vi "Ranger Dashboard.vi"() -> ()   [LabVIEW 2012, in "Party_Program.exe.lvrbt"]
doc: "This VI is designed to control TETRIX motors and visualize sensor data from your TETRIX Ranger Robot. Verify that your robot is configured as shown in the Schematic Editor. If you reconfigure your TETRIX Ranger Robot, change the ports in this VI and the Schematic Editor."
uses:
  Party_Program.exe.lvrbt
  <vilib>/NXT/Hardware/Plugins/Tetrix DC Motor/TetrixDCMotorAddress.ctl
  <vilib>/NXT/Block Support/NXT_InputPort.ctl
  <vilib>/NXT/Dual Mode Library/Display/drawText.vi
  <vilib>/NXT/Dual Mode Library/Sensors/Sonar_cm.vi
  <vilib>/NXT/Dual Mode Library/Sensors/Color_Detector.vi
  <vilib>/NXT/Dual Mode Library/Sensors/Touch_Pressed.vi
  <vilib>/NXT/NXTIO Xnodes/NXTIONodeSubVIs/TETRIX IO Move DC Motors.vi
  <vilib>/NXT/NXTIO Xnodes/NXTIONodeSubVIs/TETRIX IO Check Battery.vi
  <vilib>/NXT/NXTIO Xnodes/NXTIONodeSubVIs/TETRIX IO Stop DC Motors.vi
  <vilib>/NXT/NXTIO Xnodes/AddressXNode/NXTIOAddress.xnode
  <vilib>/NXT/NXTIO Xnodes/NXTIOXNode/NXTIO.xnode
  <vilib>/NXT/Subs/LVHSConnector.ctl
  <vilib>/NXT/LegoClasses/BrickReference/BrickReference.lvclass
panel:
  out "Yes / No":bool
  out "Detected Color":i16
  in  "Stop":bool
  out "TETRIX Battery Voltage":sgl(slide) scale=0.0..100.0
  in  "Right Wheel":i8(slide) scale=-100.0..100.0
  in  "Left Wheel":i8(slide) scale=-100.0..100.0
  out "Ultrasonic Sensor Data":i16(graph)
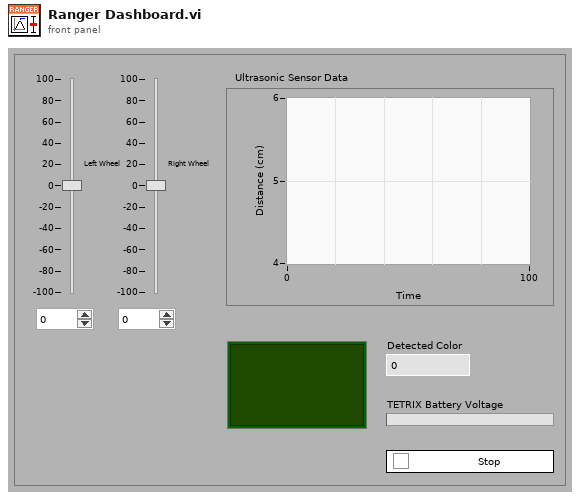
[diagram p1: front panel]
types:
  T1 = typedef "LVHSConnector.ctl" = refnum<class "BrickReference.lvclass">
  T2 = typedef "TetrixDCMotorAddress.ctl" = i16
  T3 = typedef "NXT_InputPort.ctl" = u8
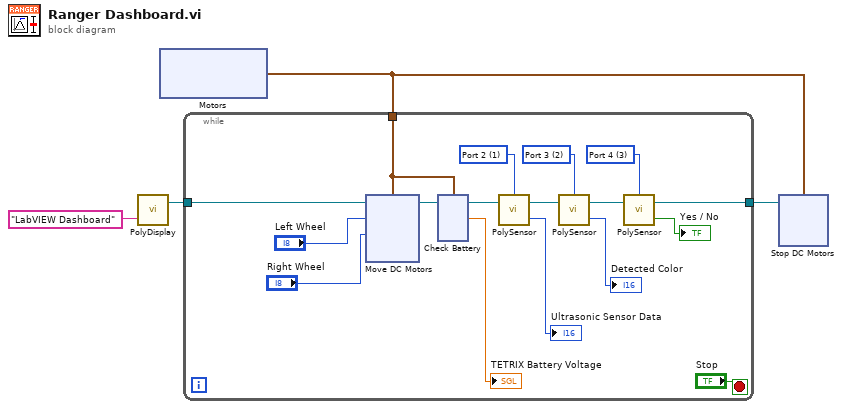
[diagram p0: block diagram]
diagram:
  n1 = call-poly <vilib>:"PolyDisplay.vi"("Text"="LabVIEW Dashboard") -> ("NXT"=w3:T1)  [unwired: 3 in]
  n2 = xnode "Motors"() -> ("Motor"=w2:cluster{"TetrixDCMotor":T2, "TetrixDCMotor":T2})
  n3 = while {
    tunnel: [w7] -> w4
    tunnel: w3 -> [w6]
    tunnel: w2 -> [w5]
    stop <- "Stop" stop-if-true
    w15 = T3 3 items=["Port 1", "Port 2", "Port 3", "Port 4"] ("Port (Port 4)")
    w16 = T3 2 items=["Port 1", "Port 2", "Port 3", "Port 4"] ("Port (Port 4)")
    w19 = T3 1 items=["Port 1", "Port 2", "Port 3", "Port 4"] ("Port (Port 4)")
    n4 = xnode "Move DC Motors"("Power/Speed 2"="Right Wheel", "Power/Speed 1"="Left Wheel", "Motors"=w5, "NXT"=w6) -> ("NXT"=w12:T1)
    n5 = xnode "Check Battery"("Motors"=w5, "NXT"=w12) -> ("Voltage 1"=→"TETRIX Battery Voltage":sgl, "NXT"=w10:T1)  [unwired: 1 out]
    n6 = call-poly <vilib>:"PolySensor.vi"("NXT"=w10, "Port (Port 4)"=w19) -> ("Distance (cm)"=→"Ultrasonic Sensor Data":i16, "NXT"=w9:T1)  [unwired: 1 in]
    n7 = call-poly <vilib>:"PolySensor.vi"("NXT"=w9, "Port (Port 3)"=w16) -> ("Detected Color"=→"Detected Color":i16, "NXT"=w8:T1)  [unwired: 1 in]
    n8 = call-poly <vilib>:"PolySensor.vi"("NXT"=w8, "Port (Port 1)"=w15) -> ("Yes / No"=→"Yes / No":bool, "NXT"=w7:T1)  [unwired: 1 in]
  }
  n9 = xnode "Stop DC Motors"("Motors"=w2, "NXT"=w4) -> ()  [unwired: 1 out]
